vi "SFOAE-Options Dialog.vi"(10 "SFOAE":T1) -> (2 "StimGen out":T1, 3 "Cancelled?":bool=TRUE)   [LabVIEW 2020]
doc: "Use this template to create a dialog box with event handling."
uses:
  Typedefs/SFOAE-Parameters.ctl
  Typedefs/SFOAE-Stimulus Parameters.ctl
  Typedefs/SFOAE-Sweep Params.ctl
  Typedefs/SFOAE-Response Parameters.ctl
panel:
  in  "Drain (ms)":dbl
  in  "Ramp (ms)":dbl
  in  "Sampling rate (Hz)":dbl
  in  "Cancel":bool
  in  "OK":bool
  # "Stimulus Parameters"
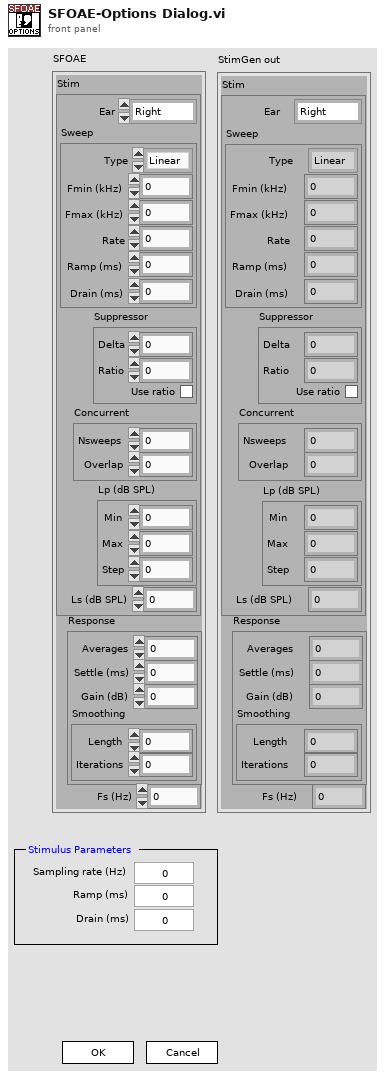
[diagram p1: front panel]
types:
  T1 = typedef "SFOAE-Parameters.ctl" = cluster{"Stim":T2, "Response":T4, "Fs (Hz)":dbl}
  T2 = typedef "SFOAE-Stimulus Parameters.ctl" = cluster{"Ear":enum16{"Right", "Left"}, "Sweep":T3, "Suppressor":cluster{"Delta":dbl, "Ratio":dbl, "Use ratio":bool}, "Concurrent":cluster{"Nsweeps":i32, "Overlap":dbl}, "Ls (dB SPL)":dbl, "Lp (dB SPL)":cluster{"Min":dbl, "Max":dbl, "Step":dbl}}
  T3 = typedef "SFOAE-Sweep Params.ctl" = cluster{"Type":enum16{"Linear", "Log"}, "Fmin (kHz)":dbl, "Fmax (kHz)":dbl, "Rate":dbl, "Ramp (ms)":dbl, "Drain (ms)":dbl}
  T4 = typedef "SFOAE-Response Parameters.ctl" = cluster{"Averages":i32, "Settle (ms)":dbl, "Gain (dB)":dbl, "Smoothing":cluster{"Length":i32, "Iterations":i32}}
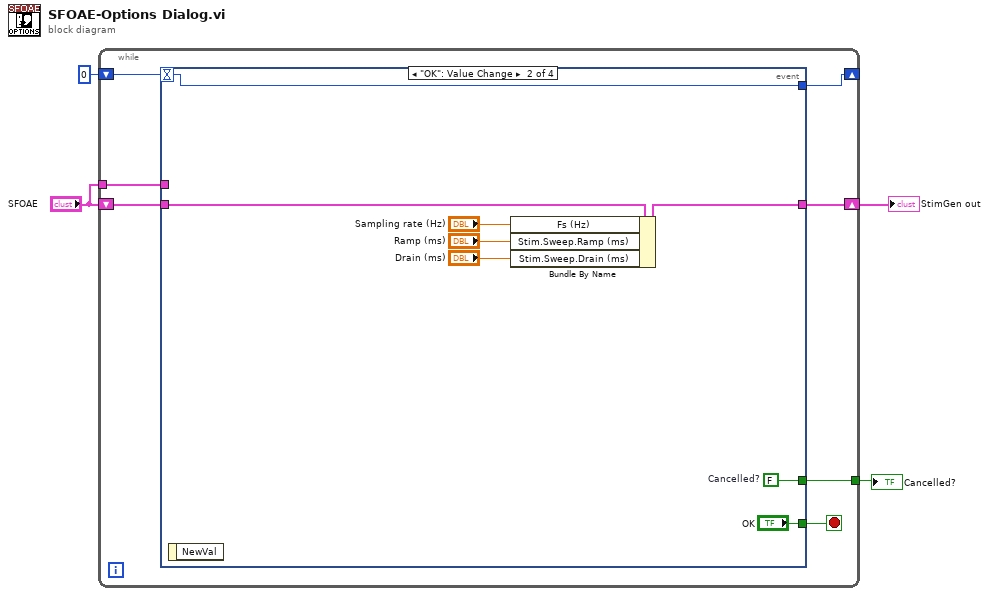
[diagram p0: block diagram]
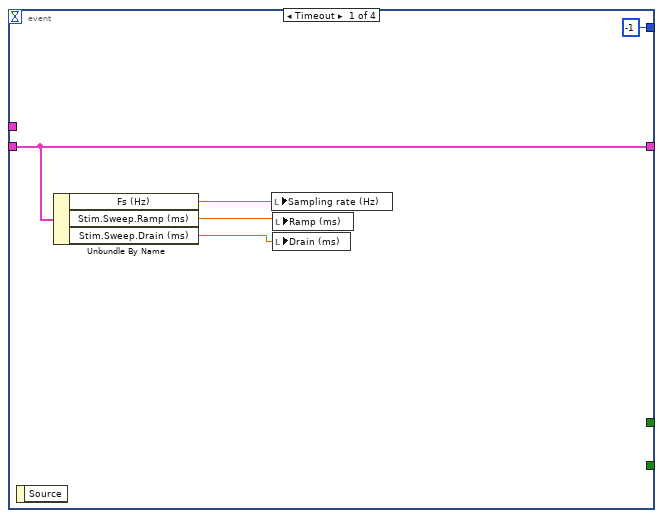
[diagram p2: hidden frame]
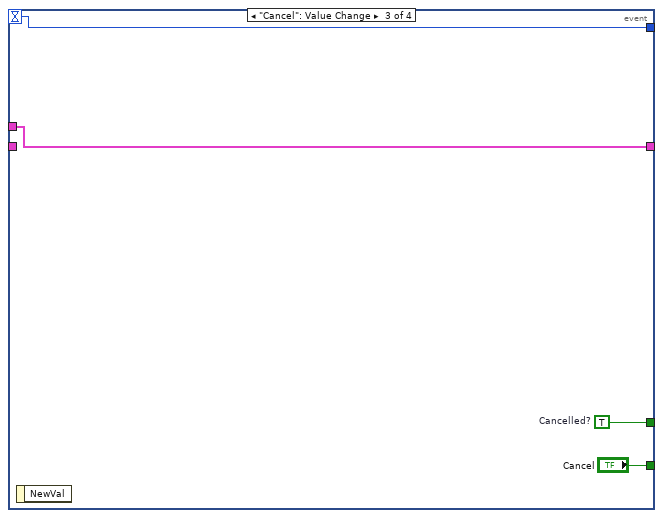
[diagram p3: hidden frame]
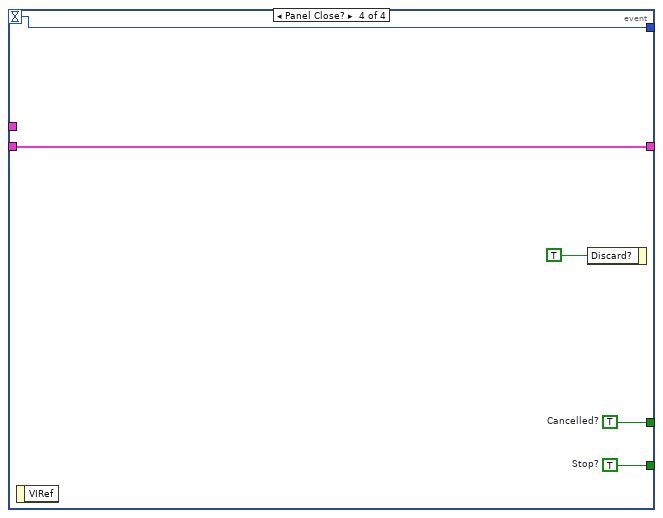
[diagram p4: hidden frame]
diagram:
  n1 = while {
    tunnel: [w10] -> w4
    shift-right: [w8] -> _
    shift-left: 0 -> [w9]
    tunnel: "SFOAE" -> [w5]
    shift-right: [w6] -> w2
    shift-left: "SFOAE" -> [w7]
    stop <- w11 stop-if-true
    n2 = event shown="[1] \"OK\": Value Change" {
      selector: _ -> [_ _ _ _]
      dyn-events: _ -> [_ _ _ _]
      timeout: w9 -> [_ w22 w26 w30]
      tunnel: [_ "OK" "Cancel" w32] -> w11
      tunnel: [_ w24 w28 w31] -> w10
      tunnel: [-1 w22 w26 w30] -> w8
      tunnel: w7 -> [w14 w21 _ w29]
      tunnel: [w14 w20 w25 w29] -> w6
      tunnel: w5 -> [_ _ w25 _]
      event Timeout {
        n3 = event-data() -> ()  [unwired: 1 in, 1 out]
        n4 = Unbundle By Name(w14) -> ("Fs (Hz)"=w15:dbl, "Stim.Sweep.Ramp (ms)"=w13:dbl, "Stim.Sweep.Drain (ms)"=w12:dbl)
        n5 = local write "Sampling rate (Hz)"(w15) -> ()
        n6 = local write "Ramp (ms)"(w13) -> ()
        n7 = local write "Drain (ms)"(w12) -> ()
      }
      event "OK": Value Change {
        w24 = FALSE  # Cancelled?
        n8 = event-data() -> ()  [unwired: 1 in, 1 out]
        n9 = Bundle By Name(cluster=w21, "Fs (Hz)"="Sampling rate (Hz)", "Stim.Sweep.Ramp (ms)"="Ramp (ms)", "Stim.Sweep.Drain (ms)"="Drain (ms)") -> (w20:T1)
      }
      event "Cancel": Value Change {
        w28 = TRUE  # Cancelled?
        n10 = event-data() -> ()  [unwired: 1 in, 1 out]
      }
      event Panel Close? {
        w31 = TRUE  # Cancelled?
        w32 = TRUE  # Stop?
        n11 = event-data() -> ()  [unwired: 1 in, 1 out]
        n12 = event-data("Discard?"=TRUE) -> ()  [unwired: 1 in, 1 out]
      }
    }
  }
  "Cancelled?" <- w4
  "StimGen out" <- w2
